vi "엔코드 속도(RPS) 측정_ 선형.vi"() -> ()   [LabVIEW 2014]
uses:
  <vilib>/DAQmx/create/channels.llb/DAQmx Create Channel (CI-Position-Linear Encoder).vi
  <vilib>/DAQmx/read.llb/DAQmx Read (Counter DBL 1Chan 1Samp).vi
panel:
  out "RPS":dbl
  out "data":dbl caption="데이터" format="%0.2f"
  in  "정지":bool
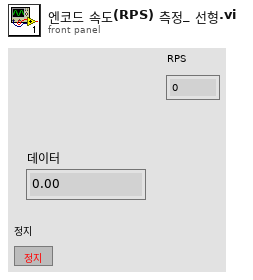
[diagram p1: front panel]
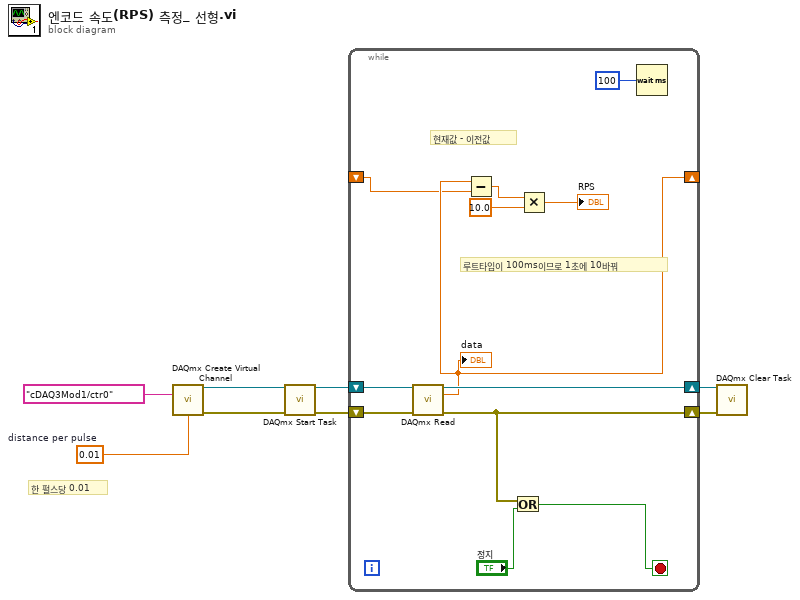
[diagram p0: block diagram]
diagram:
  w1 = 0.01  # distance per pulse
  # "한 펄스당 0.01"
  n1 = call-poly <vilib>:"DAQmx Create Virtual Channel.vi"("counter"=tag "cDAQ3Mod1/ctr0", "distance per pulse"=w1) -> ("task out"=w7:refnum<k21>, "error out"=w6:errorcluster)  [unwired: 12 in]
  n2 = call <vilib>:"DAQmx Start Task.vi"("task/channels in"=w7, "error in"=w6) -> ("task out"=w5:refnum<k21>, "error out"=w4:errorcluster)  [unwired: 12 in]
  n3 = while {
    shift-right: [w18] -> w3
    shift-left: w5 -> [w20]
    shift-right: [w16] -> w2
    shift-left: w4 -> [w19]
    shift-right: [w13] -> _
    shift-left: _ -> [w12]
    stop <- w14 stop-if-true
    # "루트타임이 100ms이므로 1초에 10바꿔"
    # "현재값 - 이전값"
    n4 = call-poly <vilib>:"DAQmx Read.vi"("task/channels in"=w20, "error in"=w19) -> ("task out"=w18:refnum<k21>, "data"=w13:dbl, "error out"=w16:errorcluster)  [unwired: 11 in]
    "data" <- w13
    n5 = Subtract(x=w13, y=w12) -> (x-y=w11:dbl)
    n6 = Or(x=w16, y="정지") -> (x .or. y?=w14:bool)
    n7 = Multiply(x=w11, y=10.0) -> (x*y=→"RPS":dbl)
    n8 = Wait (ms)(milliseconds to wait=u32 100 ("ms 배수")) -> ()  [unwired: 1 out]
  }
  n9 = call <vilib>:"DAQmx Clear Task.vi"("task in"=w3, "error in"=w2) -> ()  [unwired: 13 in, 1 out]
